vi "Operate.vi"(8 "Error In":errorcluster, 11 "Subtract In":refnum<class "Subtract.lvclass">) -> (0 "Error Out":errorcluster, 2 "C":dbl, 3 "Subtract Out":refnum<class "Subtract.lvclass">)   [LabVIEW 2021, in "Calculator.lvlib" / "Subtract.lvclass"]
doc: "This VI is an overriding method which performs the subtraction operation."
uses:
  Subtract.lvclass
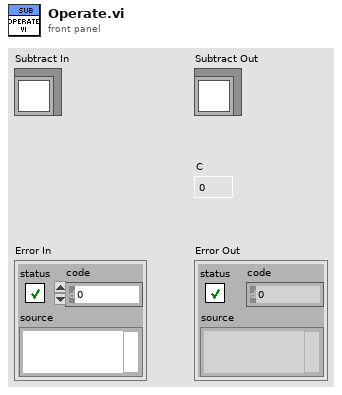
[diagram p1: front panel]
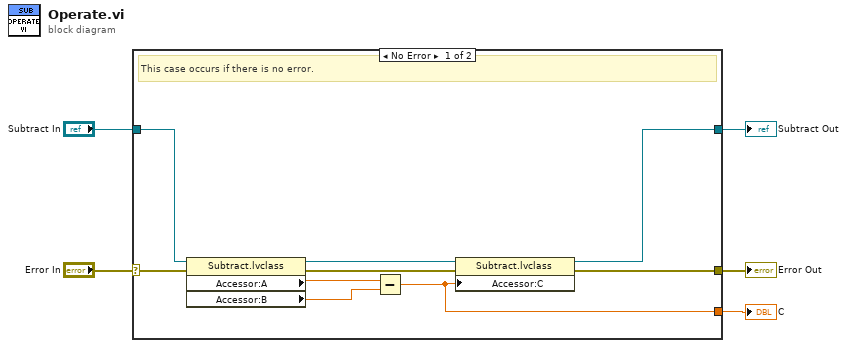
[diagram p0: block diagram]
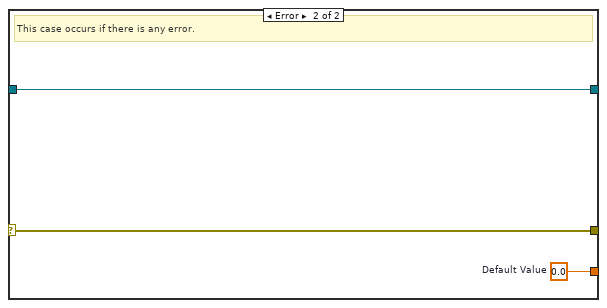
[diagram p2: hidden frame]
diagram:
  n1 = case shown="No Error" "Error In" {
    selector: "Error In" -> [w14 w17]
    tunnel: [w10 w17] -> w4
    tunnel: [w8 w16] -> w2
    tunnel: "Subtract In" -> [w7 w16]
    tunnel: [w6 w15] -> w1
    frame No Error {
      # "This case occurs if there is no error."
      n2 = property class="Subtract.lvclass"(reference=w7, error in=w14) -> (reference out=w9:refnum<class "Subtract.lvclass">, error out=w13:errorcluster, "Accessor:A"=w12:dbl, "Accessor:B"=w11:dbl)
      n3 = Subtract(x=w12, y=w11) -> (x-y=w6:dbl)
      n4 = property class="Subtract.lvclass"(reference=w9, error in=w13, "Accessor:C"=w6) -> (reference out=w8:refnum<class "Subtract.lvclass">, error out=w10:errorcluster)
    }
    frame Error {
      w15 = 0.0  # Default Value
      # "This case occurs if there is any error."
    }
  }
  "Error Out" <- w4
  "Subtract Out" <- w2
  "C" <- w1
